vi "Ejer 4.vi"() -> ()   [LabVIEW 2020]
uses:
  <vilib>/DAQmx/write.llb/DAQmx Write (Analog 1D DBL 1Chan NSamp).vi
  <vilib>/DAQmx/create/channels.llb/DAQmx Create Channel (AO-Voltage-Basic).vi
  <vilib>/DAQmx/miscellaneous.llb/DAQmx Fill In Error Info.vi
  <vilib>/measure/NI_MABase.lvlib
panel:
  in  "amplitude":dbl=2.0 format="%#_13g"
  in  "offset":dbl=-1.0 format="%#_13g"
  in  "frequency":dbl=10.0 format="%0.2p"
  out "Waveform Graph":waveform(dbl)(graph)
  in  "Stop":bool
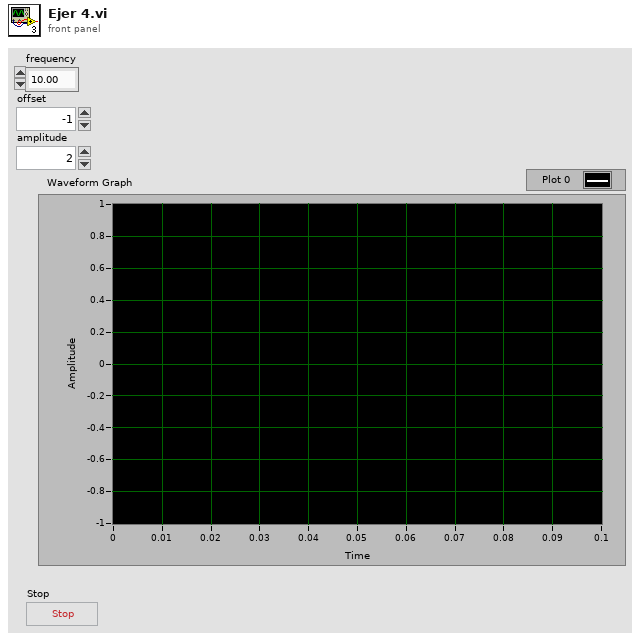
[diagram p1: front panel]
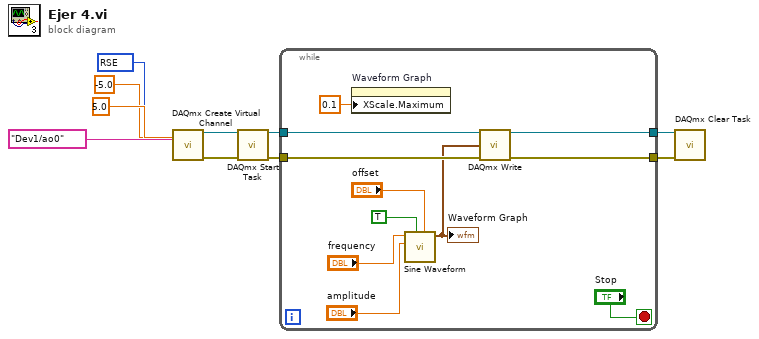
[diagram p0: block diagram]
diagram:
  w8 = 10083 items=["Default"=-1, "RSE"=10083, "NRSE"=10078, "Differential"=10106, "Pseudodifferential"=12529] ("input terminal configuration")
  n1 = call-poly <vilib>:"DAQmx Create Virtual Channel.vi"("maximum value"=5.0, "minimum value"=-5.0, "output terminal configuration"=w8, "physical channels"=tag "Dev1/ao0") -> ("task out"=w6:refnum<k21>, "error out"=w5:errorcluster)  [unwired: 10 in]
  n2 = call <vilib>:"DAQmx Start Task.vi"("task/channels in"=w6, "error in"=w5) -> ("task out"=w4:refnum<k21>, "error out"=w3:errorcluster)  [unwired: 12 in]
  n3 = while {
    tunnel: w4 -> [w20]
    tunnel: w3 -> [w19]
    tunnel: [w15] -> w2
    tunnel: [w14] -> w1
    stop <- "Stop" stop-if-true
    n4 = property on="Waveform Graph" class="WFGraph (strict)"("XScale.Maximum"=0.1 ("X Scale.Range:Maximum")) -> ()  [unwired: 2 in, 2 out]
    n5 = call <vilib>:"Sine Waveform.vi"("offset"="offset", "reset signal"=TRUE, "amplitude"="amplitude", "frequency"="frequency") -> ("signal out"=w13:waveform(dbl))  [unwired: 6 in, 1 out]
    "Waveform Graph" <- w13
    n6 = call-poly <vilib>:"DAQmx Write.vi"("task/channels in"=w20, "data"=w13, "error in"=w19) -> ("task out"=w15:refnum<k21>, "error out"=w14:errorcluster)  [unwired: 10 in, 1 out]
  }
  n7 = call <vilib>:"DAQmx Clear Task.vi"("task in"=w2, "error in"=w1) -> ()  [unwired: 13 in, 1 out]
